vi "Flatten PDU.vi"(8 "error in (no error)":errorcluster, 11 "Modbus data unit in":refnum<class "Modbus Data Unit (PDU).lvclass">) -> (0 "error out":errorcluster, 3 "full Modbus data unit":u8[](array[numeric]))   [LabVIEW 2020, in "SubVIs.lvlib" / "Modbus Data Unit (PDU).lvclass"]
uses:
  <vilib>/Modbus/subvis/Modbus Data Unit (PDU)/Modbus Data Unit (PDU).lvclass
  <vilib>/Modbus/subvis/Modbus Data Unit (PDU)/Modbus Data Unit (PDU).lvclass/Modbus Data Unit (PDU).ctl
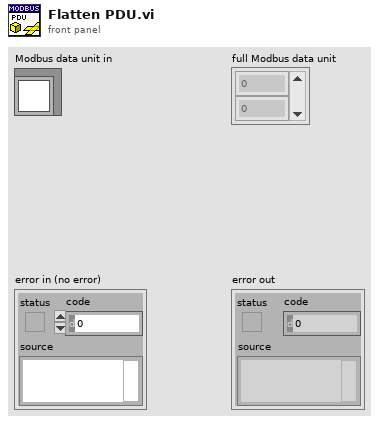
[diagram p1: front panel]
types:
  T1 = typedef "SubVIs.lvlib/Modbus Data Unit (PDU).lvclass/Function.ctl" = u8
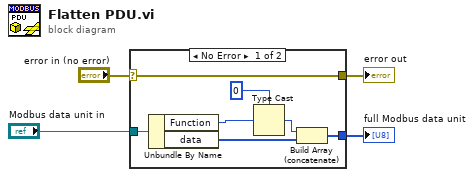
[diagram p0: block diagram]
diagram:
  n1 = case shown="No Error" "error in (no error)" {
    selector: "error in (no error)" -> [w5 w12]
    tunnel: "Modbus data unit in" -> [w11 _]
    tunnel: [w10 _] -> w3
    tunnel: [w5 w12] -> w1
    frame No Error {
      n2 = Unbundle By Name(w11) -> ("Function"=w7:T1, "data"=w6:u8[])
      n3 = Type Cast(type=u8 0, x=w7) -> (*(type *) &x=w9:u8)
      n4 = Build Array (concatenate)(w9, w6) -> (w10:u8[])
    }
    frame Error {
    }
  }
  "error out" <- w1
  "full Modbus data unit" <- w3
